vi "Periodic Tasks.vi"(8 "error in":errorcluster) -> ()   [LabVIEW 2013]
doc: "This VI runs in parallel to other tasks. It can contain as many user-defined periodic loops as you need. These can carry out PID or other sorts of timed response."
uses:
  <vilib>/Rock Robotics/SystemInterfaces/Utilities/FPGA_UtilitiesLED Source.ctl
  <vilib>/Rock Robotics/SystemInterfaces/Utilities/FPGA_UtilitiesLED State.ctl
  <vilib>/Rock Robotics/WPI/Relay/WPI_RelayValue.ctl
  <vilib>/Rock Robotics/WPI/Joystick/WPI_JoystickGetSetRefNum.vi
  Robot Global Data.vi
  <vilib>/Rock Robotics/WPI/RobotDrive/WPI_RobotDriveGetSetRefNum.vi
  <vilib>/Rock Robotics/WPI/Compressor/WPI_CompressorGetSetRefNum.vi
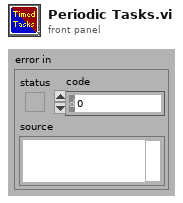
[diagram p1: front panel]
types:
  T1 = typedef "FPGA_UtilitiesLED State.ctl" = enum16{"Off", "On", "Toggle"}
  T2 = typedef "FPGA_UtilitiesLED Source.ctl" = enum16{"User LED", "FPGA LED"}
  T3 = typedef "WPI_CompressorDevRef.ctl" = cluster{"DevStatus":errorcluster, "DigitalInputDevRef":T4, "RelayDevRef":T7}
  T4 = typedef "WPI_DigitalInputDevRef.ctl" = cluster{"DevStatus":errorcluster, "DIO Channel":T5, "Digital Module":T6}
  T5 = typedef "FPGA_DIOChannel.ctl" = enum8{"DIO 1", "DIO 2", "DIO 3", "DIO 4", "DIO 5", "DIO 6", "DIO 7", "DIO 8", "DIO 9", "DIO 10", "DIO 11", "DIO 12", "DIO 13", "DIO 14", "Invalid"}
  T6 = typedef "FPGA_TypedefDigitalModule.ctl" = enum16{"Digital Module 1", "Digital Module 2"}
  T7 = typedef "WPI_RelayDevRef.ctl" = cluster{"DevStatus":errorcluster, "Relay Channel":T8, "Digital Module":T6, "Relay Direction":T9}
  T8 = typedef "FPGA_DIORelayChannel.ctl" = enum8{"Relay 1", "Relay 2", "Relay 3", "Relay 4", "Relay 5", "Relay 6", "Relay 7", "Relay 8", "Invalid"}
  T9 = typedef "WPI_RelayDirection.ctl" = enum16{"Both directions", "Forward only", "Reverse only"}
  T10 = typedef "WPI_RobotDriveDevRef.ctl" = cluster{"DevStatus":errorcluster, "Motors[]":T11[], "Square Inputs":bool, "Max Output":dbl, "Isochronous":bool}
  T11 = typedef "WPI_MotorControlDeviceRef.ctl" = cluster{"DeviceStatus":errorcluster, "Type":enum16{"PWM", "CAN"}, "PWM":cluster{"Digital Module":T6, "PWM Channel":T12, "DeadBand":T13}, "CAN":cluster{"Device Number":u8, "Control Mode":T14, "Semaphore":T15, "Max Vout":dbl}, "Invert":bool, "TransformRef":T16, "InvTransformRef":T16}
  T12 = typedef "FPGA_DIOPWMChannel.ctl" = enum8{"PWM 1", "PWM 2", "PWM 3", "PWM 4", "PWM 5", "PWM 6", "PWM 7", "PWM 8", "PWM 9", "PWM 10", "Invalid"}
  T13 = typedef "WPI_PWMDeadband.ctl" = cluster{"Name":string, "maxPositivePwm":i32, "minPositivePwm":i32, "centerPwm":i32, "maxNegativePwm":i32, "minNegativePwm":i32, "angularRange":u16}
  T14 = typedef "WPI_CANJaguar_ControlMode.ctl" = enum8{"Percent VBus", "Current", "Speed", "Position", "Voltage"}
  T15 = typedef "Semaphore RefNum" = refnum<k1>
  T16 = typedef "WPI_PWMTransform_ConPane.ctl" = refnum<vi>
  T17 = typedef "WPI_JoystickDevRef.ctl" = cluster{"Device":T18}
  T18 = typedef "WPI_JoystickDeviceEnum.ctl" = enum16{"USB 1", "USB 2", "USB 3", "USB 4", "Kinect 1", "Kinect 2"}
  T19 = cluster{"JoystickDevRef":T17, "RobotDriveDevRef":T10}
  T20 = typedef "WPI_JoystickButtonState.ctl" = cluster{"Button 1":bool, "Button 2":bool, "Button 3":bool, "Button 4":bool, "Button 5":bool, "Button 6":bool, "Button 7":bool, "Button 8":bool, "Button 9":bool, "Button 10":bool, "Button 11":bool, "Button 12":bool}
  T21 = typedef "WPI_RelayValue.ctl" = enum16{"Off", "On", "Forward", "Reverse"}
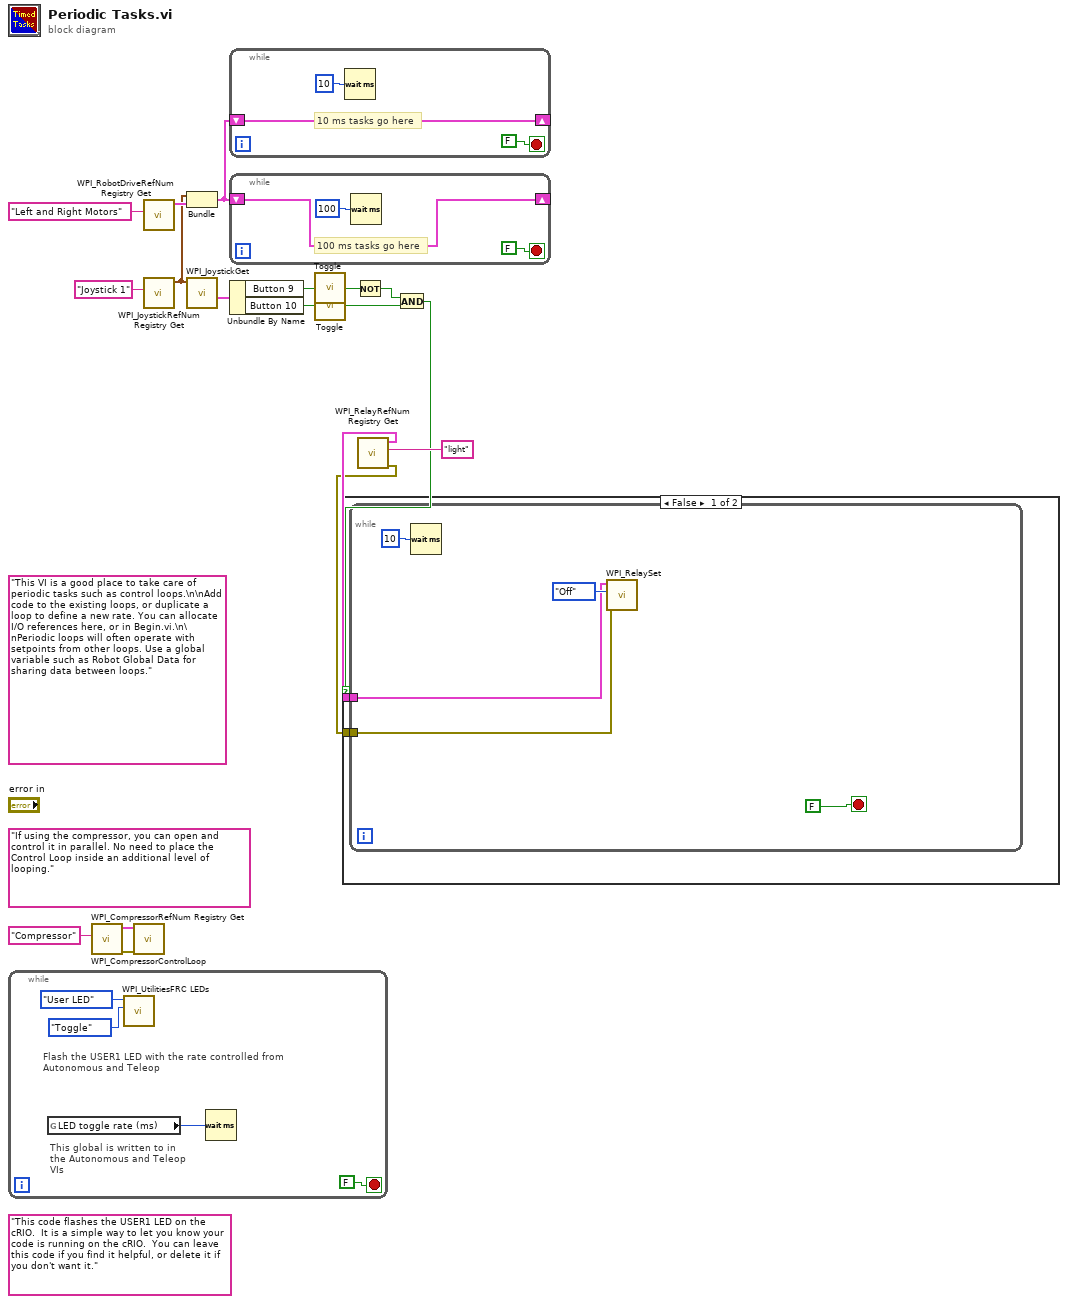
[diagram p0: block diagram]
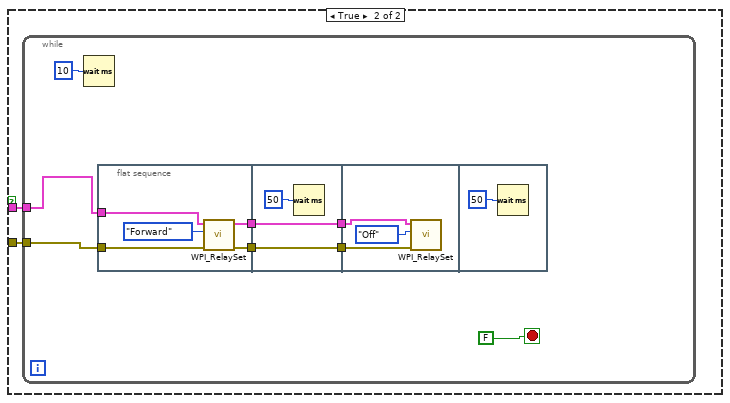
[diagram p2: hidden frame]
diagram:
  (unwired) "If using the compressor, you can open and control it in parallel. No need to place the Control Loop inside an additional level of looping."
  (unwired) "This code flashes the USER1 LED on the cRIO.  It is a simple way to let you know your code is running on the cRIO.  You can leave this code if you find it helpful, or delete it if you don't want it."
  (unwired) "This VI is a good place to take care of periodic tasks such as control loops.\n\nAdd code to the existing loops, or duplicate a loop to define a new rate. You can allocate I/O references here, or in Begin.vi.\n\nPeriodic loops will often operate with setpoints from other loops. Use a global variable such as Robot Global Data for sharing data between loops."
  n1 = while {
    stop <- FALSE stop-if-true
    # "This global is written to in the Autonomous and Teleop VIs"
    # "Flash the USER1 LED with the rate controlled from Autonomous and Teleop"
    n2 = global read "Robot Global Data.vi" "LED toggle rate (ms)"() -> (w19:u32)
    n3 = call <vilib>:"WPI_UtilitiesFRC LEDs.vi"("State"=FPGA_UtilitiesLED_State."Toggle", "LED Type"=FPGA_UtilitiesLED_Source."User LED") -> ()  [unwired: 1 in, 9 out]
    n4 = Wait (ms)(milliseconds to wait=w19) -> ()  [unwired: 1 out]
  }
  n5 = call <vilib>:"WPI_CompressorRefNum Registry Get.vi"("refnum name"="Compressor") -> ("error out"=w16:errorcluster, "CompressorDevRef"=w17:T3)  [unwired: 9 in]
  n6 = call <vilib>:"WPI_CompressorControlLoop.vi"("error in (no error)"=w16, "CompressorDevRef"=w17) -> ()  [unwired: 10 in]
  n7 = call <vilib>:"WPI_RobotDriveRefNum Registry Get.vi"("refnum name"="Left and Right Motors") -> ("RobotDriveDevRef"=w13:T10)  [unwired: 1 in, 9 out]
  n8 = call <vilib>:"WPI_JoystickRefNum Registry Get.vi"("refnum name"="Joystick 1") -> ("JoystickDevRef"=w11:T17)  [unwired: 1 in, 9 out]
  n9 = Bundle("JoystickDevRef"=w11, "RobotDriveDevRef"=w13) -> (w12:T19)  [unwired: 1 out]
  n10 = call <vilib>:"WPI_JoystickGet.vi"("JoystickDevRef"=w11) -> ("Buttons"=w4:T20)  [unwired: 1 in, 5 out]
  n11 = while {
    shift-right: [w23] -> _
    shift-left: w12 -> [w23]
    stop <- FALSE stop-if-true
    # "10 ms tasks go here"
    n12 = Wait (ms)(milliseconds to wait=u32 10) -> ()  [unwired: 1 out]
  }
  n13 = while {
    shift-right: [w26] -> _
    shift-left: w12 -> [w26]
    stop <- FALSE stop-if-true
    # "100 ms tasks go here"
    n14 = Wait (ms)(milliseconds to wait=u32 100) -> ()  [unwired: 1 out]
  }
  n15 = Unbundle By Name(w4) -> ("Button 9"=w8:bool, "Button 10"=w7:bool)
  n16 = call "Toggle.vi"("Input"=w8) -> ("Output"=w9:bool)
  n17 = call "Toggle.vi"("Input"=w7) -> ("Output"=w6:bool)
  n18 = Not(x=w9) -> (.not. x?=w10:bool)
  n19 = call <vilib>:"WPI_RelayRefNum Registry Get.vi"("refnum name"="light") -> ("error out"=w2:errorcluster, "RelayDevRef"=w3:T7)  [unwired: 9 in]
  n20 = And(x=w10, y=w6) -> (x .and. y?=w1:bool)
  n21 = case shown="False" w1 {
    tunnel: w3 -> [w30 w37]
    tunnel: w2 -> [w29 w36]
    frame False {
      n22 = while {
        tunnel: w30 -> [w32]
        tunnel: w29 -> [w31]
        stop <- FALSE stop-if-true
        n23 = Wait (ms)(milliseconds to wait=u32 10) -> ()  [unwired: 1 out]
        n24 = call <vilib>:"WPI_RelaySet.vi"("error in (no error)"=w31, "RelayValue"=WPI_RelayValue."Off", "RelayDevRef"=w32) -> ()  [unwired: 7 in, 2 out]
      }
    }
    frame True {
      n25 = while {
        tunnel: w37 -> [w43]
        tunnel: w36 -> [w42]
        stop <- FALSE stop-if-true
        n26 = Wait (ms)(milliseconds to wait=u32 10) -> ()  [unwired: 1 out]
        n27 = flat-sequence {
          tunnel: [w50] -> w41
          tunnel: [w49] -> w40
          tunnel: w43 -> [w47]
          tunnel: w42 -> [w46]
          tunnel: [w52] -> w39
          tunnel: w41 -> [w52]
          tunnel: [w51] -> w38
          tunnel: w40 -> [w51]
          tunnel: w39 -> [w56]
          tunnel: w38 -> [w55]
          frame #0 {
            n28 = call <vilib>:"WPI_RelaySet.vi"("error in (no error)"=w46, "RelayValue"=WPI_RelayValue."Forward", "RelayDevRef"=w47) -> ("error out"=w49:errorcluster, "RelayDevRef"=w50:T7)  [unwired: 7 in]
          }
          frame #1 {
            n29 = Wait (ms)(milliseconds to wait=u32 50) -> ()  [unwired: 1 out]
          }
          frame #2 {
            n30 = call <vilib>:"WPI_RelaySet.vi"("error in (no error)"=w55, "RelayValue"=WPI_RelayValue."Off", "RelayDevRef"=w56) -> ()  [unwired: 7 in, 2 out]
          }
          frame #3 {
            n31 = Wait (ms)(milliseconds to wait=u32 50) -> ()  [unwired: 1 out]
          }
        }
      }
    }
  }
